vi "CreateChildCore.vi"(10 "InnerLocalConfig":T1, 11 "ChildConfig":T1) -> ()   [LabVIEW 2020, in "jettl.lvlib"]
uses:
  jettl.lvlib
  Actor Layer/Actor Layer.lvclass
  Config.ctl
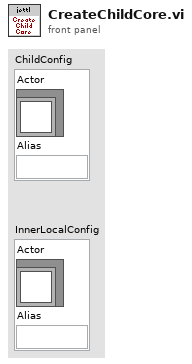
[diagram p1: front panel]
types:
  T1 = typedef "jettl.lvlib/Config.ctl" = cluster{"Actor":refnum<class "Actor Layer.lvclass">, "Alias":string}
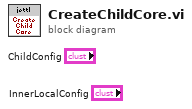
[diagram p0: block diagram]
diagram:
